vi "Import Dialog.vi"(8 "error in":errorcluster, 11 "Item Ref in":T1 format="%.0x") -> (0 "error out":errorcluster, 3 "Item Ref out":T1 format="%.0x")   [LabVIEW 2019, in "DSF System Explorer.lvlib"]
doc: "Implements the import dialog for DSF configuration"
uses:
  DSF System Explorer.lvlib
  DSF Core.lvlibp/Typedefs/DSF Timing Info.ctl
  DSF Core.lvlibp/Typedefs/Core Plugin Configuration.ctl
  DSF Core.lvlibp/Typedefs/DSF Settings Info.ctl
  DSF Core.lvlibp/Typedefs/Core Thread Configuration.ctl
  DSF Core.lvlibp/Typedefs/DSF Direction.ctl
  DSF Core.lvlibp/Typedefs/DSF Timeout Behavior.ctl
  DSF Core.lvlibp/Typedefs/Core Group Configuration.ctl
  DSF Core.lvlibp/Typedefs/Core Transfer Configuration.ctl
  DSF Core.lvlibp/Typedefs/DSF Data Type.ctl
  DSF Core.lvlibp/Typedefs/Core Channel Configuration.ctl
  DSF Core.lvlibp/Typedefs/DSF Engine Channel Configuration.ctl
  DSF Core.lvlibp/Typedefs/DSF Engine Transfer Configuration.ctl
  DSF Core.lvlibp/Typedefs/DSF Engine Transfer Group Configuration.ctl
  DSF Core.lvlibp/Typedefs/DSF Engine Plugin Thread Configuration.ctl
  DSF Core.lvlibp/Typedefs/DSF Engine Plugin Configuration.ctl
  DSF Core.lvlibp/Typedefs/DSF Engine Framework Configuration.ctl
  <vilib>/NI VeriStand/Custom Device API/Custom Device Item Ref.ctl
  <vilib>/NI VeriStand/Custom Device API/Custom Device API.lvlib
panel:
  out "Duration":u32 format="%d ms"
  out "Version":string
  in  "Apply":bool
  in  "Load":bool
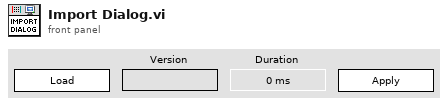
[diagram p1: front panel]
types:
  T1 = typedef "Custom Device API.lvlib/Custom Device Item Ref.ctl" = u64
  T2 = typedef "DSF Core.lvlibp/DSF Engine Framework Configuration.ctl" = cluster{"plugins":T3[]}
  T3 = typedef "DSF Core.lvlibp/DSF Engine Plugin Configuration.ctl" = cluster{"core":T4, "component settings":T6[], "threads":T7[]}
  T4 = typedef "DSF Core.lvlibp/Plugin Configuration.lvclass/Core Plugin Configuration.ctl" = cluster{"name":string, "components":string[], "cycle timing":T5}
  T5 = typedef "DSF Core.lvlibp/DSF Timing Info.ctl" = cluster{"priority":u64, "decimation":u64, "offset":u64}
  T6 = typedef "DSF Core.lvlibp/DSF Settings Info.ctl" = cluster{"component":string, "values":cluster{"key":string, "value":string}[]}
  T7 = typedef "DSF Core.lvlibp/DSF Engine Plugin Thread Configuration.ctl" = cluster{"core":T8, "component settings":T6[], "transfer groups":T9[]}
  T8 = typedef "DSF Core.lvlibp/Thread Configuration.lvclass/Core Thread Configuration.ctl" = cluster{"processor":i32, "priority offset":i16}
  T9 = typedef "DSF Core.lvlibp/DSF Engine Transfer Group Configuration.ctl" = cluster{"core":T10, "component settings":T6[], "transfers":T13[]}
  T10 = typedef "DSF Core.lvlibp/Group Configuration.lvclass/Core Group Configuration.ctl" = cluster{"name":string, "direction":T11, "cycle timing":T5, "timeout behavior":T12, "enable conversion":bool}
  T11 = typedef "DSF Core.lvlibp/DSF Direction.ctl" = enum8{"Tx", "Rx"}
  T12 = typedef "DSF Core.lvlibp/DSF Timeout Behavior.ctl" = enum8{"Increment Late Count", "Throw Error"}
  T13 = typedef "DSF Core.lvlibp/DSF Engine Transfer Configuration.ctl" = cluster{"core":T14, "component settings":T6[], "channels":T15[]}
  T14 = typedef "DSF Core.lvlibp/Transfer Configuration.lvclass/Core Transfer Configuration.ctl" = cluster{"name":string}
  T15 = typedef "DSF Core.lvlibp/DSF Engine Channel Configuration.ctl" = cluster{"core":T16, "component settings":T6[]}
  T16 = typedef "DSF Core.lvlibp/Channel Configuration.lvclass/Core Channel Configuration.ctl" = cluster{"name":string, "units":string, "engine data type":T17, "string data type":T17, "string offset":u64}
  T17 = typedef "DSF Core.lvlibp/DSF Data Type.ctl" = enum8{"Bool", "SGL", "DBL", "I8", "I16", "I32", "I64", "U8", "U16", "U32", "U64"}
  T18 = enum8{"Enabled", "Disabled", "Disabled and Grayed Out"}
  T19 = typedef "DSF Core.lvlibp/DSF Version Info.ctl" = cluster{"major":u32, "minor":u32, "fix":u32, "build":string}
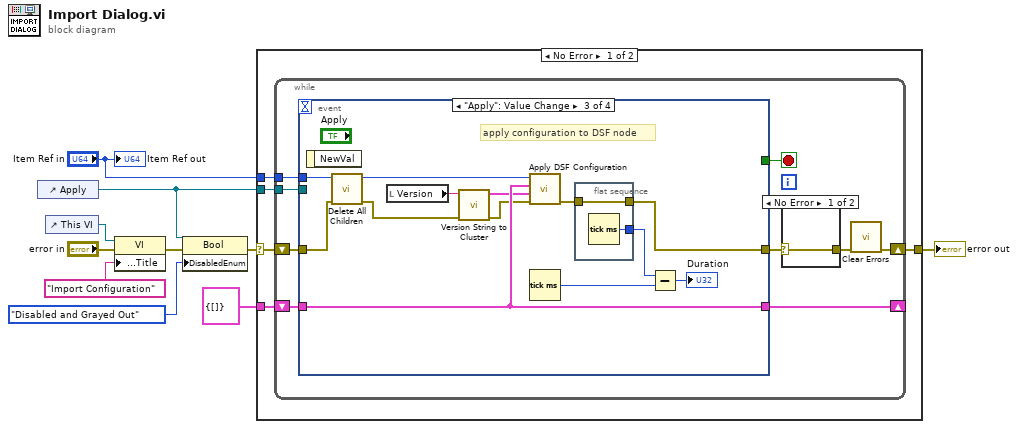
[diagram p0: block diagram]
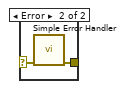
[diagram p2: hidden frame]
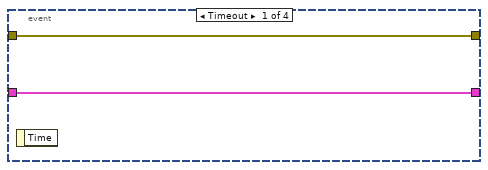
[diagram p3: hidden frame]
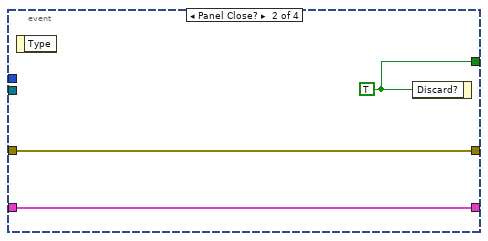
[diagram p4: hidden frame]
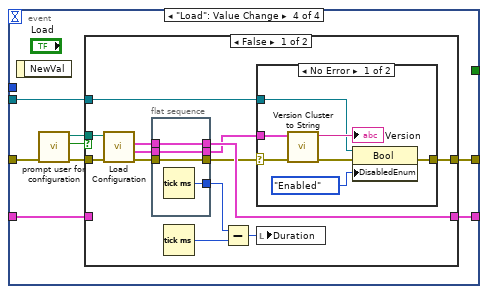
[diagram p5: hidden frame]
diagram:
  n1 = control-ref of="Apply"() -> (w3:refnum<vi>)
  n2 = control-ref of="This VI"() -> (w9:refnum<vi>)
  n3 = property class="VI"(reference=w9, error in="error in", "Front Panel.Title"="Import Configuration" ("Front Panel Window:Title")) -> (error out=w5:errorcluster)  [unwired: 1 out]
  n4 = property class="Bool"(reference=w3, error in=w5, "DisabledEnum"=T18."Disabled and Grayed Out" ("Disabled")) -> (error out=w4:errorcluster)  [unwired: 1 out]
  n5 = case shown="No Error" w4 {
    selector: w4 -> [w11 w83]
    tunnel: [w15 w83] -> w10
    tunnel: "Item Ref in" -> [w14 _]
    tunnel: w3 -> [w13 _]
    tunnel: T2 {"plugins"=[]} ("framework configuration") -> [w12 _]
    frame No Error {
      n6 = while {
        tunnel: w14 -> [w18]
        shift-right: [w20] -> _
        shift-left: w12 -> [w19]
        tunnel: w13 -> [w17]
        shift-right: [w23] -> w15
        shift-left: w11 -> [w16]
        stop <- w24 stop-if-true
        n7 = event shown="[2] \"Apply\": Value Change" {
          selector: _ -> [_ _ _ _]
          dyn-events: _ -> [_ _ _ _]
          timeout: _ -> [_ _ _ _]
          tunnel: [_ w31 _ _] -> w24
          tunnel: [w28 w30 w34 w50] -> w22
          tunnel: w18 -> [_ _ w40 _]
          tunnel: w19 -> [w29 w32 w45 w52]
          tunnel: [w29 w32 w45 w55] -> w20
          tunnel: w17 -> [_ _ _ w49]
          tunnel: w16 -> [w28 w30 w35 w48]
          event Timeout {
            n8 = event-data() -> ()  [unwired: 1 in, 1 out]
          }
          event Panel Close? {
            w31 = TRUE ("Discard?")
            n9 = event-data() -> ()  [unwired: 1 in, 1 out]
            n10 = event-data("Discard?"=w31) -> ()  [unwired: 1 in, 1 out]
          }
          event "Apply": Value Change {
            # "apply configuration to DSF node"
            n11 = event-data() -> ()  [unwired: 1 in, 1 out]
            n12 = call "Delete All Children.vi"("error in (no error)"=w35, "Item Ref in"=w40) -> ("error out"=w39:errorcluster, "Item Ref out"=w44:T1)  [unwired: 8 in]
            n13 = local read "Version"() -> (w43:string)
            n14 = call "Version String to Cluster.vi"("error in (no error)"=w39, "version string"=w43) -> ("error out"=w42:errorcluster, "version"=w41:T19)  [unwired: 8 in]
            n15 = call "Apply DSF Configuration.vi"("error in (no error)"=w42, "version"=w41, "framework configuration"=w45, "Item Ref in"=w44) -> ("error out"=w33:errorcluster)  [unwired: 7 in]
            n16 = Tick Count (ms)() -> (millisecond timer value=w36:u32)
            n17 = flat-sequence {
              tunnel: [w47] -> w38
              tunnel: [w46] -> w34
              tunnel: w33 -> [w46]
              frame #0 {
                n18 = Tick Count (ms)() -> (millisecond timer value=w47:u32)
              }
            }
            n19 = Subtract(x=w38, y=w36) -> (x-y=→"Duration":u32)
          }
          event "Load": Value Change {
            n20 = event-data() -> ()  [unwired: 1 in, 1 out]
            n21 = call "prompt user for configuration.vi"("error in (no error)"=w48) -> ("error out"=w54:errorcluster, "cancelled"=w51:bool, "selected path"=w53:path)  [unwired: 8 in]
            n22 = case shown="False" w51 {
              tunnel: [w66 w81] -> w50
              tunnel: [w61 w82] -> w55
              tunnel: w54 -> [w68 w81]
              tunnel: w53 -> [w67 _]
              tunnel: w52 -> [_ w82]
              tunnel: w49 -> [w62 _]
              frame False {
                n23 = call "Load Configuration.vi"("error in (no error)"=w68, "configuration file path"=w67) -> ("error out"=w56:errorcluster, "version"=w58:T19, "framework configuration"=w60:T2)  [unwired: 6 in, 1 out]
                n24 = flat-sequence {
                  tunnel: [w72] -> w65
                  tunnel: [w71] -> w61
                  tunnel: w60 -> [w71]
                  tunnel: [w70] -> w59
                  tunnel: w58 -> [w70]
                  tunnel: [w69] -> w57
                  tunnel: w56 -> [w69]
                  frame #0 {
                    n25 = Tick Count (ms)() -> (millisecond timer value=w72:u32)
                  }
                }
                n26 = Tick Count (ms)() -> (millisecond timer value=w63:u32)
                n27 = Subtract(x=w65, y=w63) -> (x-y=w64:u32)
                n28 = case shown="No Error" w57 {
                  selector: w57 -> [w77 w80]
                  tunnel: [w73 w80] -> w66
                  tunnel: w59 -> [w76 _]
                  tunnel: w62 -> [w75 _]
                  frame No Error {
                    n29 = call "Version Cluster to String.vi"("error in (no error)"=w77, "version"=w76) -> ("error out"=w74:errorcluster, "version string"=→"Version":string)  [unwired: 8 in]
                    n30 = property class="Bool"(reference=w75, error in=w74, "DisabledEnum"=T18."Enabled" ("Disabled")) -> (error out=w73:errorcluster)  [unwired: 1 out]
                  }
                  frame Error {
                  }
                }
                n31 = local write "Duration"(w64) -> ()
              }
              frame True {
              }
            }
          }
        }
        n32 = case shown="No Error" w22 {
          selector: w22 -> [w25 w27]
          tunnel: [w25 w26] -> w21
          frame No Error {
          }
          frame Error {
            n33 = call <vilib>:"Simple Error Handler.vi"("error in (no error)"=w27) -> ("error out"=w26:errorcluster)  [unwired: 4 in, 4 out]
          }
        }
        n34 = call <vilib>:"Clear Errors.vi"("error in (no error)"=w21) -> ("error out"=w23:errorcluster)  [unwired: 5 in, 1 out]
      }
    }
    frame Error {
    }
  }
  "error out" <- w10
  "Item Ref out" <- "Item Ref in"
